vi "ProjInitialize.vi"(8 "error in (no error)":errorcluster, 11 "CS++MessageMakerMain in":refnum<class "CS++MessageMakerMain.lvclass">) -> (0 "error out":errorcluster, 3 "CS++MessageMakerMain out":refnum<class "CS++MessageMakerMain.lvclass">)   [LabVIEW 2015, in "CS++MessageMakerMain.lvlib" / "CS++MessageMakerMain.lvclass"]
doc: "Initialize a specific Project. This VI loads Actor Objects, Method Objects and Message Objects."
uses:
  CS++MessageMakerMain.lvclass
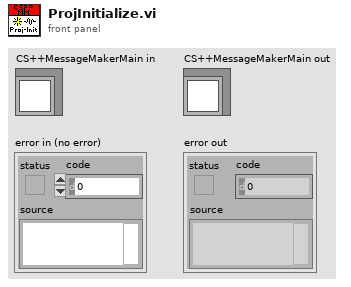
[diagram p1: front panel]
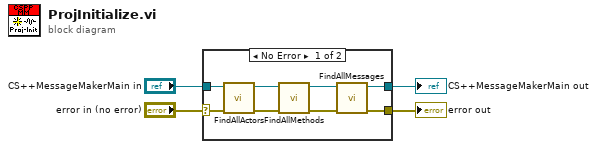
[diagram p0: block diagram]
diagram:
  n1 = case shown="No Error" "error in (no error)" {
    selector: "error in (no error)" -> [w11 w14]
    tunnel: [w5 w14] -> w3
    tunnel: [w6 w13] -> w1
    tunnel: "CS++MessageMakerMain in" -> [w12 w13]
    frame No Error {
      n2 = call "FindAllActors.vi"("error in (no error)"=w11, "CS++MessageMakerMain in"=w12) -> ("error out"=w10:errorcluster, "CS++MessageMakerMain out"=w9:refnum<class "CS++MessageMakerMain.lvclass">)  [unwired: 8 in]
      n3 = call "FindAllMethods.vi"("error in (no error)"=w10, "CS++MessageMakerMain in"=w9) -> ("error out"=w8:errorcluster, "CS++MessageMakerMain out"=w7:refnum<class "CS++MessageMakerMain.lvclass">)  [unwired: 8 in]
      n4 = call "FindAllMessages.vi"("error in (no error)"=w8, "CS++MessageMakerMain in"=w7) -> ("error out"=w5:errorcluster, "CS++MessageMakerMain out"=w6:refnum<class "CS++MessageMakerMain.lvclass">)  [unwired: 8 in]
    }
    frame Error {
    }
  }
  "error out" <- w3
  "CS++MessageMakerMain out" <- w1
